vi "test microFPGA VIs SL.vi"() -> ()   [LabVIEW 2016]
panel:
  in  "write or read":u16(ring)=1 items=["read", "write"]
  out "analog value read":i32
  out "value write confirm 5":bool
  out "value write confirm 4":bool
  out "value confirm":bool
  out "value write confirm 3":bool
  out "value write confirm 2":bool
  out "value write confirm":bool
  in  "servo position write":u32(slide)=12706 max=65535 step=1 scale=0.0..65535.0 scale format="%u us"
  out "Version":u16=1
  in  "PWM ratio":u32(slide)=49 max=255 step=1 scale=0.0..255.0 scale format="%u us"
  in  "TTL mode":u16(ring)=1 items=["LO", "HIGH"]
  in  "laser number":u16(ring) items=["laser No 0", "laser No 1", "laser No 2", "laser No 3", "laser No 4", "laser No 5"]
  in  "laser mode":u16(ring)=2 items=["OFF", "ON", "RISING", "FALLING", "CAMERA"]
  in  "sequence":bool[](array[boolean])=[TRUE, FALSE, FALSE, FALSE, FALSE, FALSE, FALSE, FALSE, FALSE, FALSE, FALSE, FALSE, FALSE, FALSE, FALSE, FALSE]
  in  "duration":u32(slide)=9 max=65535 step=1 scale=0.0..65535.0 scale format="%u us"
  in  "stop":bool=TRUE
  in  "send":bool
  # "initial readout of the version after init"
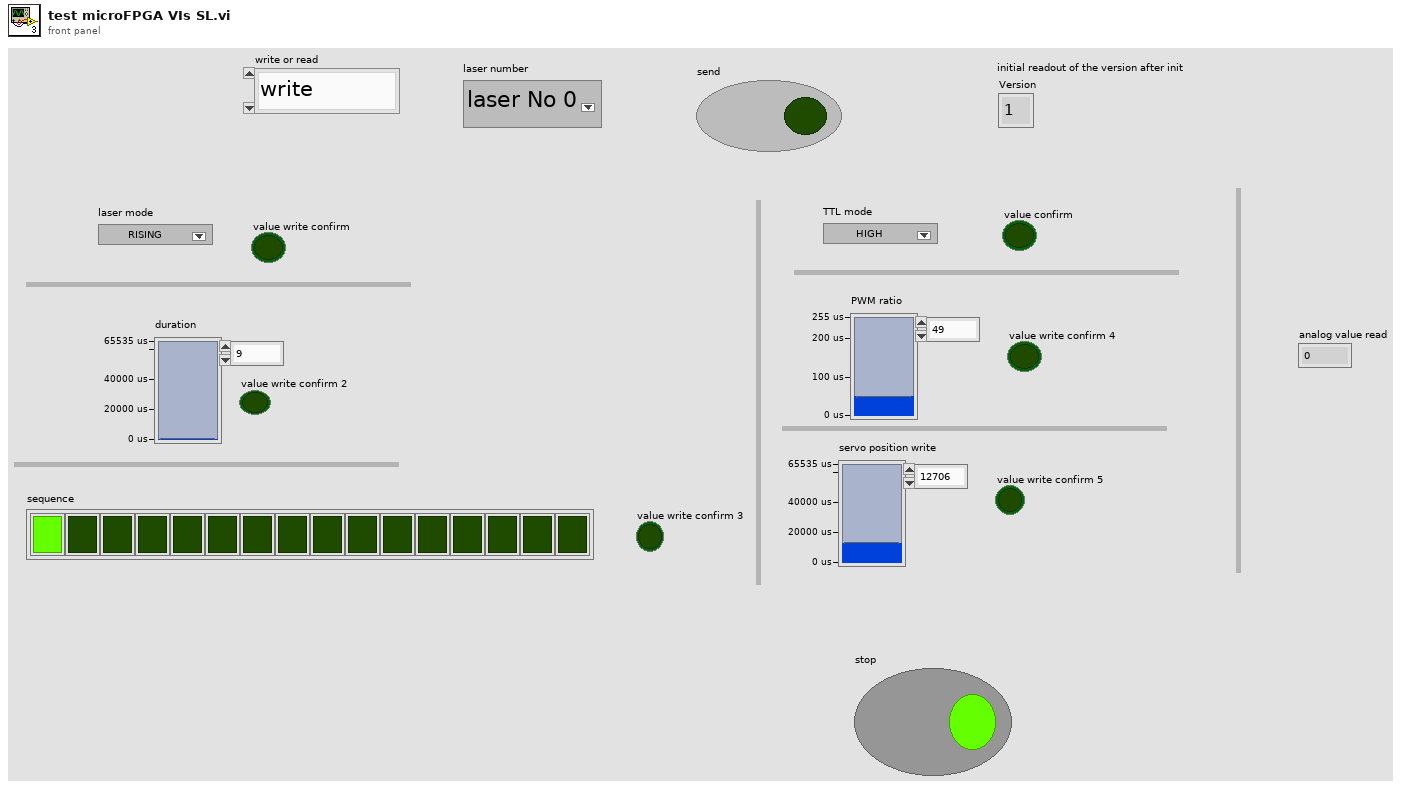
[diagram p1: front panel]
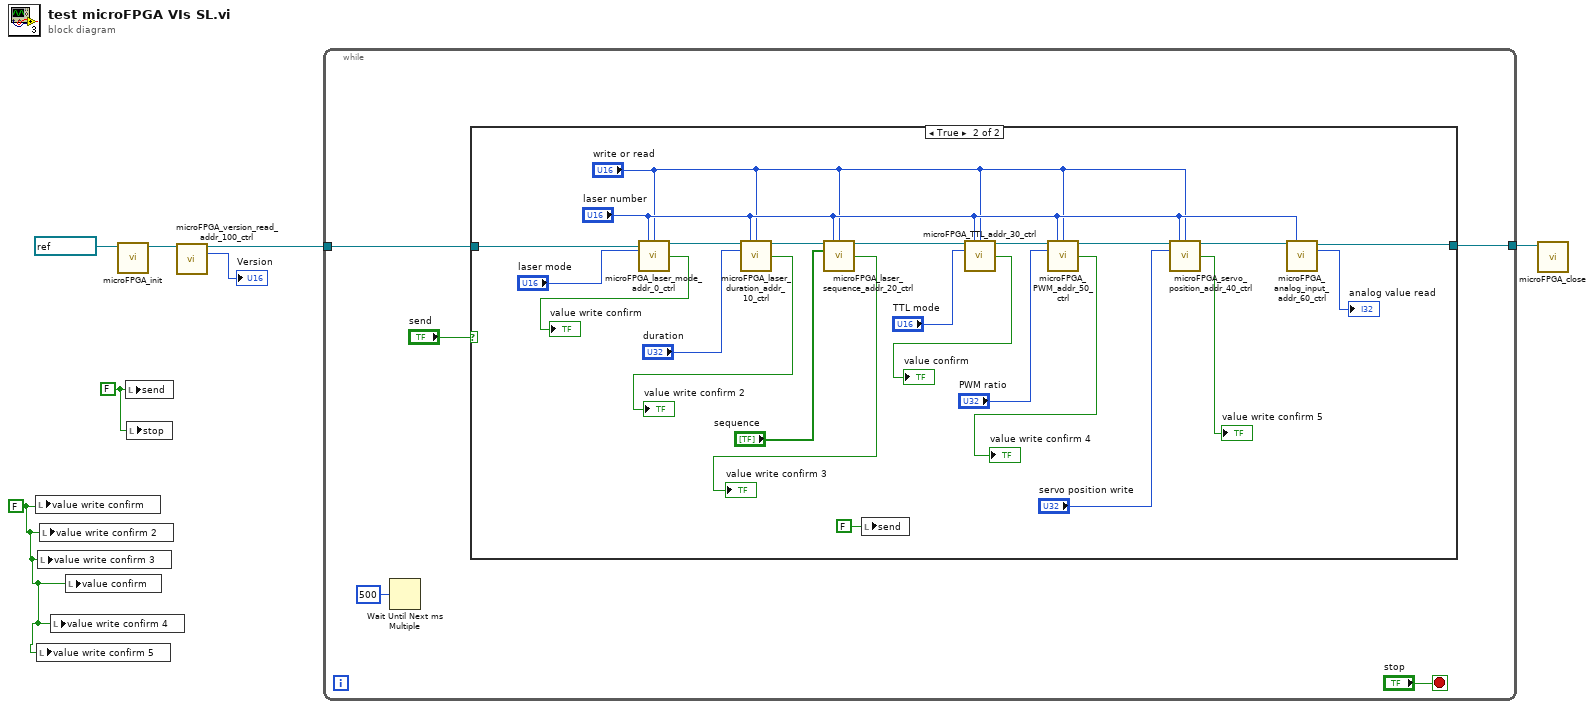
[diagram p0: block diagram]
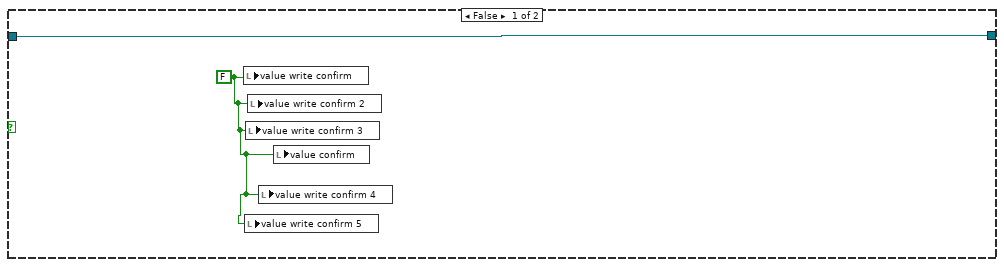
[diagram p2: hidden frame]
diagram:
  w3 = FALSE ("write")
  w7 = FALSE ("write")
  n1 = local write "value write confirm"(w3) -> ()
  n2 = local write "value write confirm 5"(w3) -> ()
  n3 = local write "value write confirm 3"(w3) -> ()
  n4 = local write "value write confirm 2"(w3) -> ()
  n5 = local write "value write confirm 4"(w3) -> ()
  n6 = local write "value confirm"(w3) -> ()
  n7 = call "microFPGA_init.vi"("VISA resource name"=refnum<visa-resource-name> "COM6") -> ("VISA resource name out"=w6:refnum<visa-resource-name>)  [unwired: 9 in, 1 out]
  n8 = local write "send"(w7) -> ()
  n9 = local write "stop"(w7) -> ()
  n10 = call "microFPGA_version_read_addr_100_ctrl.vi"("VISA resource name"=w6) -> ("VISA resource name 2"=w5:refnum<visa-resource-name>, "Version"=→"Version":u16)  [unwired: 12 in, 1 out]
  n11 = while {
    tunnel: w5 -> [w9]
    tunnel: [w8] -> w2
    stop <- "stop" stop-if-true
    n12 = Wait Until Next ms Multiple(millisecond multiple=u32 500) -> ()  [unwired: 1 out]
    n13 = case shown="True" "send" {
      tunnel: w9 -> [w13 w31]
      tunnel: [w13 w15] -> w8
      frame False {
        w14 = FALSE ("write")
        n14 = local write "value write confirm"(w14) -> ()
        n15 = local write "value write confirm 5"(w14) -> ()
        n16 = local write "value write confirm 3"(w14) -> ()
        n17 = local write "value write confirm 2"(w14) -> ()
        n18 = local write "value write confirm 4"(w14) -> ()
        n19 = local write "value confirm"(w14) -> ()
      }
      frame True {
        n20 = call "microFPGA_laser_mode_addr_0_ctrl.vi"("VISA resource name"=w31, "laser channel"="laser number", "write or read"="write or read", "laser mode write"="laser mode") -> ("VISA resource name 2"=w29:refnum<visa-resource-name>, "value write confirm"=→"value write confirm":bool)  [unwired: 7 in, 3 out]
        n21 = call "microFPGA_laser_duration_addr_10_ctrl.vi"("VISA resource name"=w29, "laser channel"="laser number", "write or read"="write or read", "duration write"="duration") -> ("VISA resource name 2"=w26:refnum<visa-resource-name>, "value write confirm"=→"value write confirm 2":bool)  [unwired: 7 in, 3 out]
        n22 = call "microFPGA_laser_sequence_addr_20_ctrl.vi"("VISA resource name"=w26, "laser channel"="laser number", "write or read"="write or read", "sequence write"="sequence") -> ("VISA resource name 2"=w25:refnum<visa-resource-name>, "value write confirm"=→"value write confirm 3":bool)  [unwired: 7 in, 3 out]
        n23 = local write "send"(FALSE ("write")) -> ()
        n24 = call "microFPGA_TTL_addr_30_ctrl.vi"("VISA resource name"=w25, "TTL channel"="laser number", "write or read"="write or read", "TTL mode"="TTL mode") -> ("VISA out"=w37:refnum<visa-resource-name>, "value confirm"=→"value confirm":bool)  [unwired: 7 in, 3 out]
        n25 = call "microFPGA_PWM_addr_50_ctrl.vi"("VISA resource name"=w37, "PWM channel"="laser number", "write or read"="write or read", "PWM ratio write"="PWM ratio") -> ("VISA resource name 2"=w34:refnum<visa-resource-name>, "value write confirm"=→"value write confirm 4":bool)  [unwired: 7 in, 3 out]
        n26 = call "microFPGA_servo_position_addr_40_ctrl.vi"("VISA resource name"=w34, "servo channel"="laser number", "write or read"="write or read", "servo position write"="servo position write") -> ("VISA resource name 2"=w33:refnum<visa-resource-name>, "value write confirm"=→"value write confirm 5":bool)  [unwired: 7 in, 3 out]
        n27 = call "microFPGA_analog_input_addr_60_ctrl.vi"("VISA resource name"=w33, "analog readout channel"="laser number") -> ("VISA resource name 2"=w15:refnum<visa-resource-name>, "analog value read"=→"analog value read":i32)  [unwired: 10 in, 2 out]
      }
    }
  }
  n28 = call "microFPGA_close.vi"("VISA resource name"=w2) -> ()  [unwired: 11 in]
